vi "getRewardStimulus.vi"(8 "error in (no error)":errorcluster, 11 "Stimulus in":refnum<class "Stimulus.lvclass">) -> (0 "error out":errorcluster, 1 "Last Juice time":timestamp, 2 "RI":dbl, 3 "Stimulus out":refnum<class "Stimulus.lvclass">, 4 "Pulse Duration":dbl)   [LabVIEW 2014, in "Stimulus.lvclass"]
uses:
  Stimulus.lvclass
  Stimulus.lvclass/Stimulus.ctl
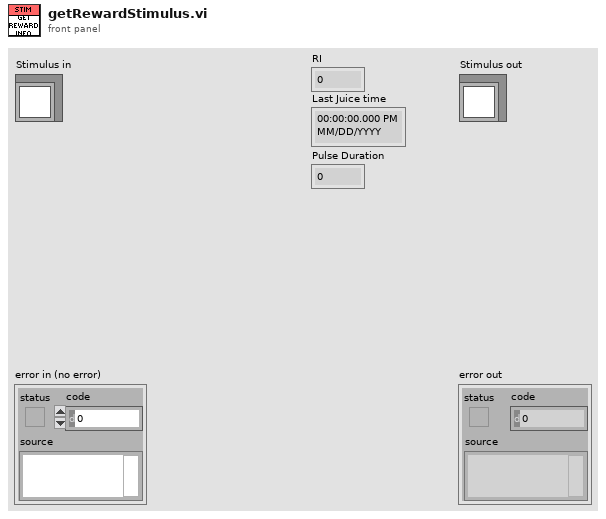
[diagram p1: front panel]
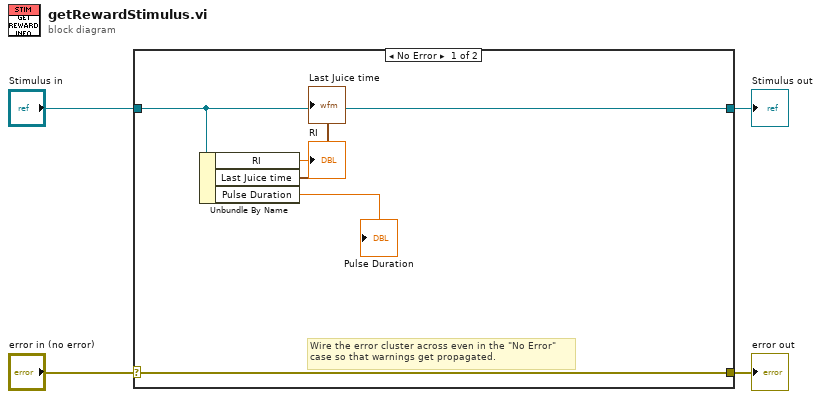
[diagram p0: block diagram]
diagram:
  n1 = case shown="No Error" "error in (no error)" {
    selector: "error in (no error)" -> [w9 w11]
    tunnel: [w9 w11] -> w3
    tunnel: [w8 w10] -> w1
    tunnel: "Stimulus in" -> [w8 w10]
    frame No Error {
      # "Wire the error cluster across even in the \"No Error\"\ncase so that warnings get propagated."
      n2 = Unbundle By Name(w8) -> ("RI"=→"RI":dbl, "Last Juice time"=→"Last Juice time":timestamp, "Pulse Duration"=→"Pulse Duration":dbl)
    }
    frame Error {
    }
  }
  "error out" <- w3
  "Stimulus out" <- w1
